vi "CREA_CLUSTER.vi"(0 "FOTOCELULA":bool, 1 "RFID_Error":errorcluster, 4 "RFID_LR6_Error":errorcluster, 6 "DC":bool, 7 "TEMPERATURA":bool, 8 "WHEEL_SENSOR":bool, 9 "all rows":dbl[][](array[numeric]), 10 "LIMITE MAX":dbl, 11 "LIMITE MIN":dbl, 12 "ERROR FPGA":errorcluster, 13 "ERROR ESCRITURA":errorcluster) -> (20 "appended array":cluster{string, dbl, "output string":string}[](array[cluster]), 22 "ESTADO WRD":dbl)   [LabVIEW 2015]
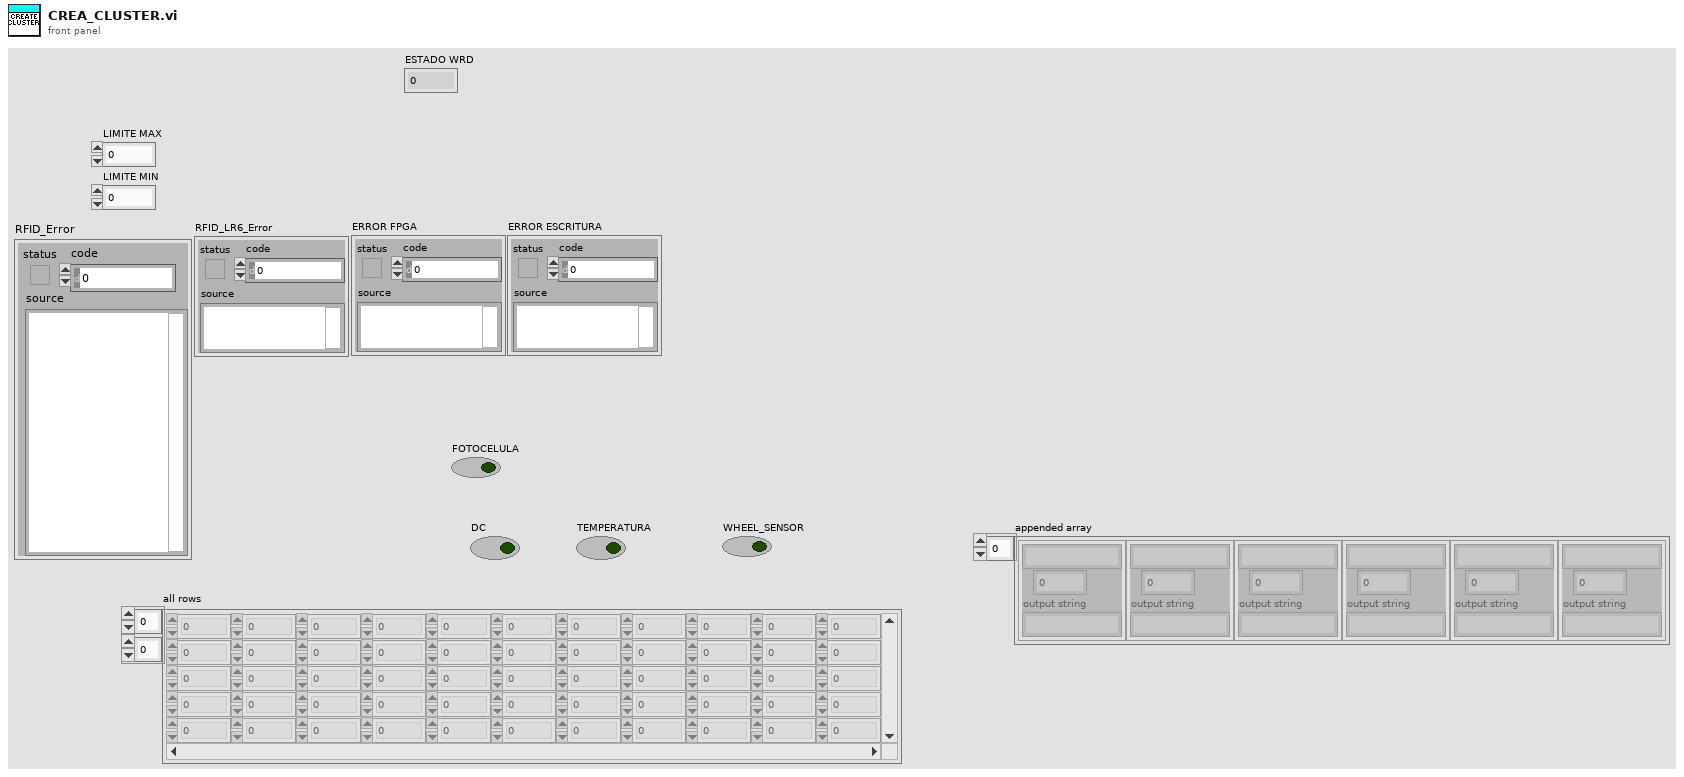
[diagram p1: front panel]
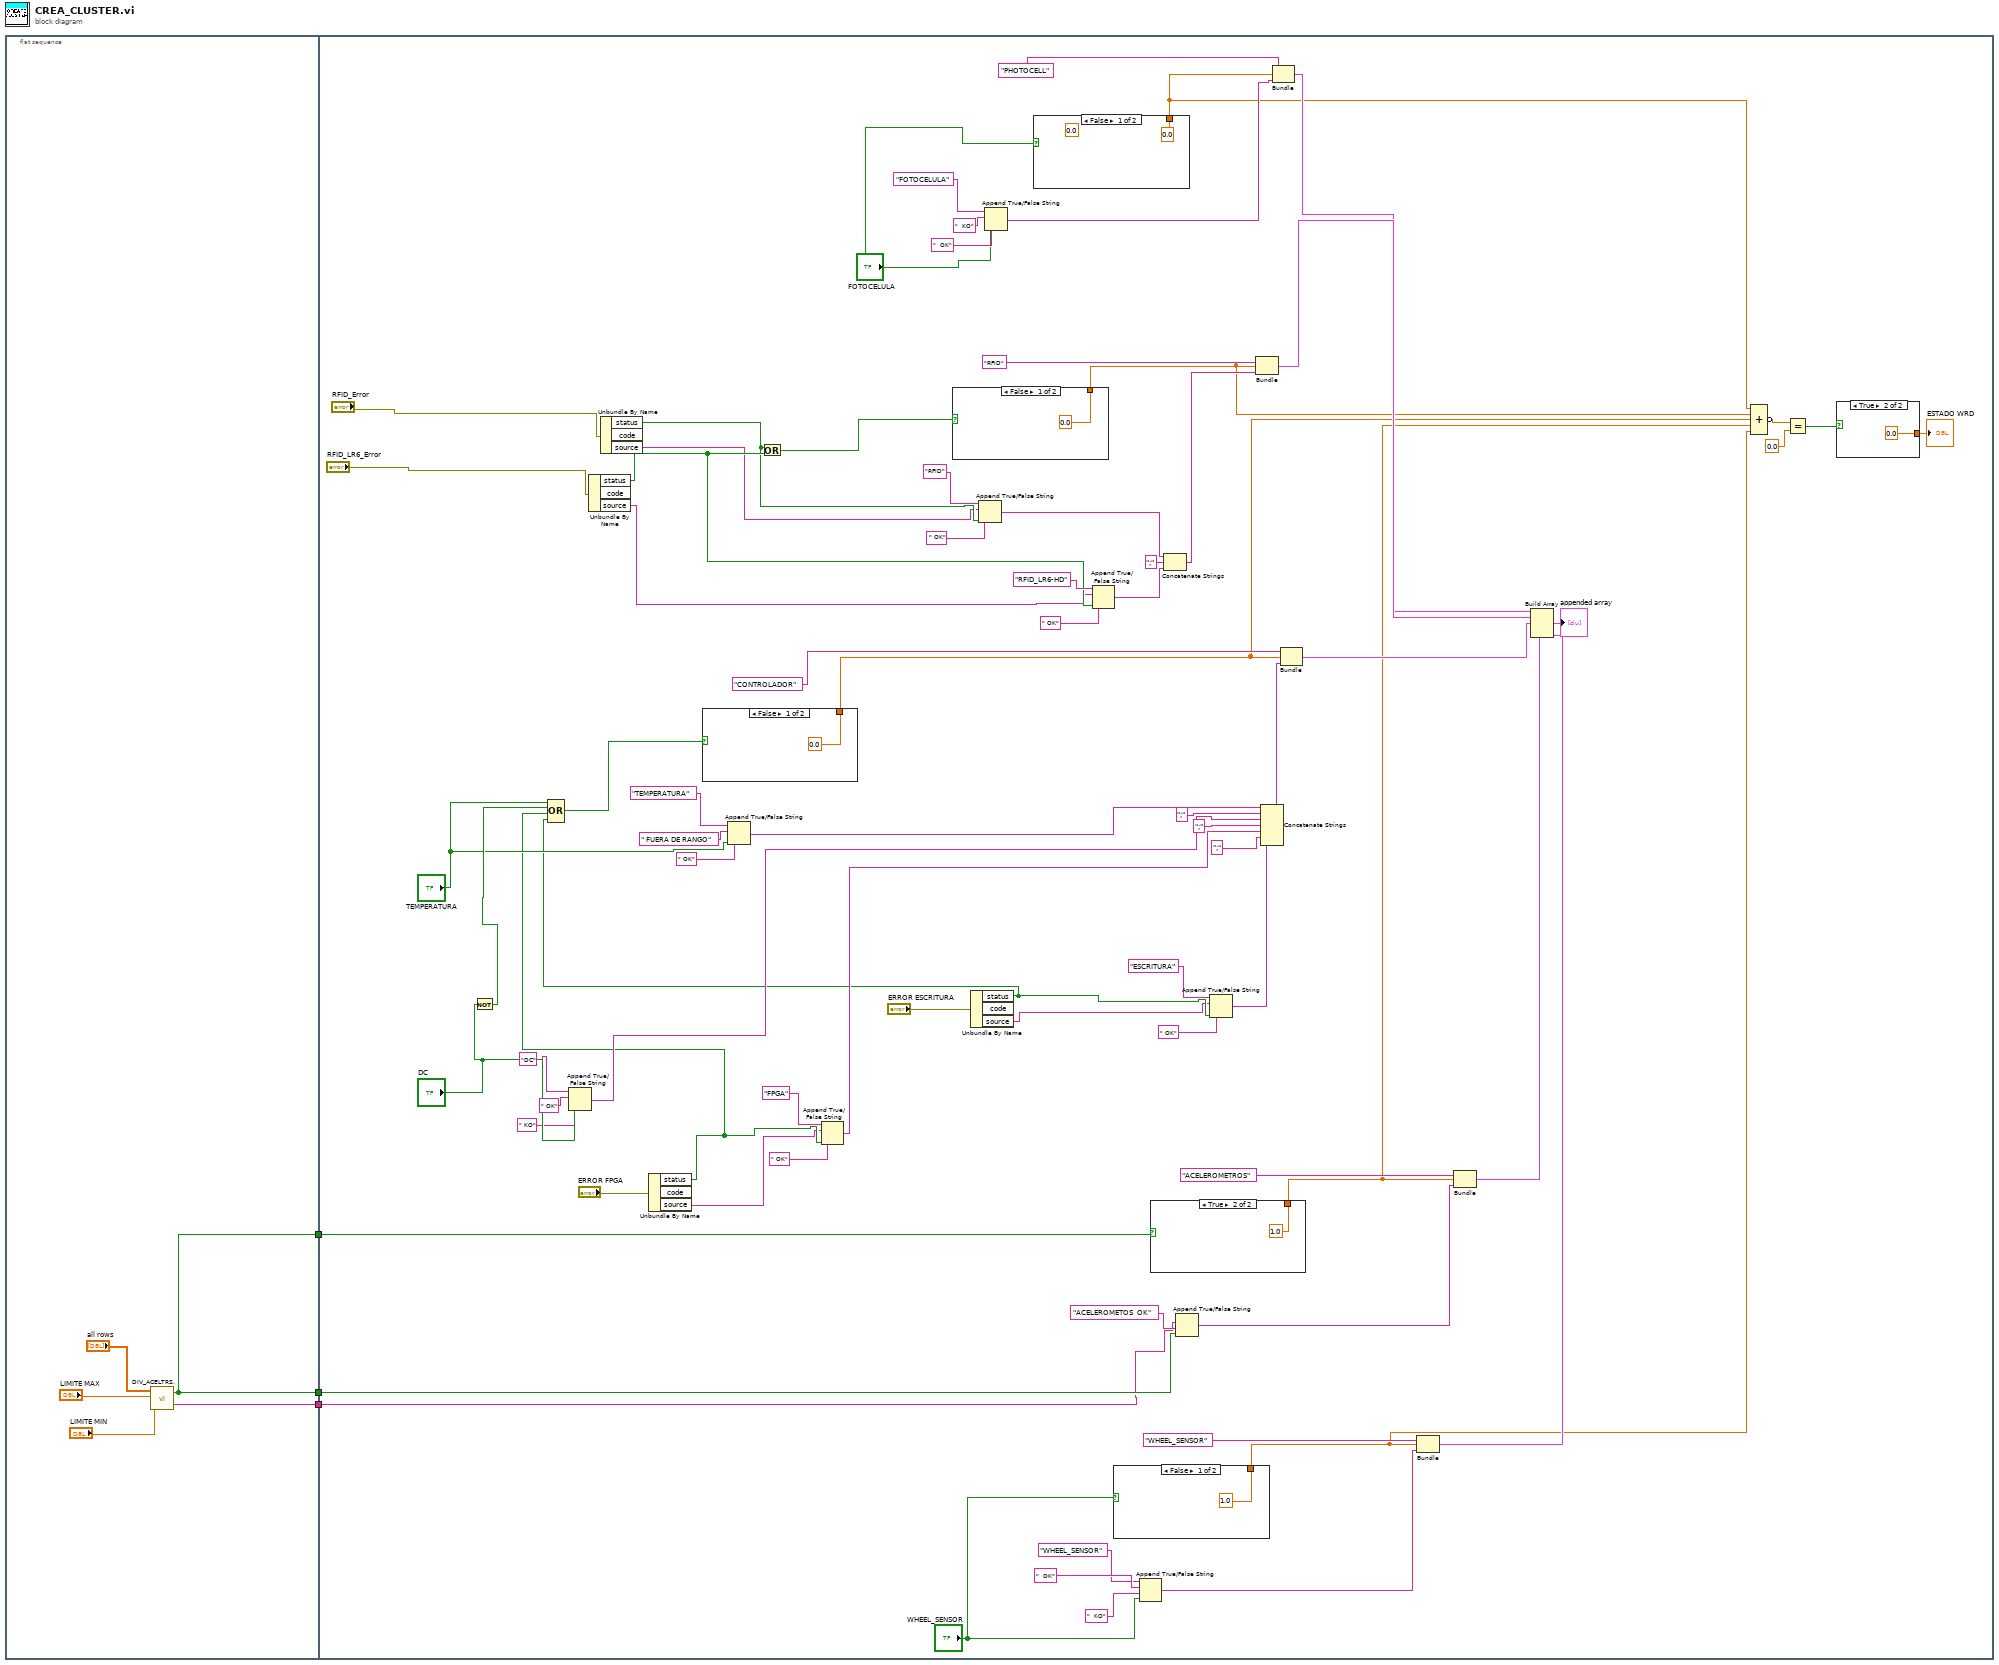
[diagram p0: block diagram]
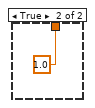
[diagram p2: hidden frame]
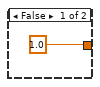
[diagram p3: hidden frame]
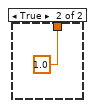
[diagram p4: hidden frame]
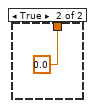
[diagram p5: hidden frame]
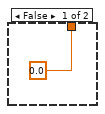
[diagram p6: hidden frame]
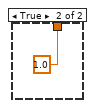
[diagram p7: hidden frame]
diagram:
  n1 = flat-sequence {
    tunnel: [w7] -> w3
    tunnel: [w6] -> w2
    tunnel: [w6] -> w1
    tunnel: w3 -> [w27]
    tunnel: w2 -> [w30]
    tunnel: w1 -> [w35]
    frame #0 {
      n2 = call "DIV_ACELTRS..vi"("LIMITE MIN 2"="LIMITE MIN", "LIMITE MAX 2"="LIMITE MAX", "all rows"="all rows") -> ("concatenated string"=w7:string, "ACELEROMETROS OK"=w6:bool)  [unwired: 3 in]
    }
    frame #1 {
      (unwired) 0.0
      n3 = Not(x="DC") -> (.not. x?=w86:bool)
      n4 = Append True/False String(1:"DC", 2:" KO" ("false string"), 3:" OK" ("true string"), 4:"DC" ("string (\"\")")) -> (0:w80:string)
      n5 = Unbundle By Name("RFID_LR6_Error") -> ("status"=w72:bool, "source"=w17:string)  [unwired: 1 out]
      n6 = Unbundle By Name("RFID_Error") -> ("status"=w71:bool, "source"=w18:string)  [unwired: 1 out]
      n7 = Unbundle By Name("ERROR FPGA") -> ("status"=w10:bool, "source"=w9:string)  [unwired: 1 out]
      n8 = Append True/False String(1:"TEMPERATURA", 2:" OK" ("false string"), 3:" FUERA DE RANGO" ("true string"), 4:"TEMPERATURA" ("string (\"\")")) -> (0:w65:string)
      n9 = Or(x=w71, y=w72) -> (x .or. y?=w73:bool)
      n10 = Append True/False String(1:w10, 2:" OK" ("false string"), 3:w9, 4:"FPGA" ("string (\"\")")) -> (0:w82:string)
      n11 = case shown="False" w73 {
        tunnel: [0.0 1.0] -> w25
        frame False {
        }
        frame True {
        }
      }
      n12 = Unbundle By Name("ERROR ESCRITURA") -> ("status"=w13:bool, "source"=w12:string)  [unwired: 1 out]
      n13 = Compound Arithmetic op=OR("TEMPERATURA", w86, w10, w13) -> (w67:bool)
      n14 = case shown="False" w67 {
        tunnel: [0.0 1.0] -> w24
        frame False {
        }
        frame True {
        }
      }
      n15 = Append True/False String(1:w71, 2:" OK" ("false string"), 3:w18, 4:"RFID" ("string (\"\")")) -> (0:w59:string)
      n16 = Append True/False String(1:"FOTOCELULA", 2:"  OK" ("false string"), 3:"  KO" ("true string"), 4:"FOTOCELULA" ("string (\"\")")) -> (0:w32:string)
      n17 = case shown="False" "FOTOCELULA" {
        tunnel: [0.0 1.0] -> w26
        frame False {
        }
        frame True {
        }
      }
      n18 = Append True/False String(1:w72, 2:" OK" ("false string"), 3:w17, 4:"RFID_LR6-HD" ("string (\"\")")) -> (0:w77:string)
      n19 = case shown="False" "WHEEL_SENSOR" {
        tunnel: [1.0 0.0] -> w22
        frame False {
        }
        frame True {
        }
      }
      n20 = Append True/False String(1:"WHEEL_SENSOR", 2:"  KO" ("false string"), 3:"  OK" ("true string"), 4:"WHEEL_SENSOR" ("string (\"\")")) -> (0:w49:string)
      n21 = case shown="True" w30 {
        tunnel: [0.0 1.0] -> w23
        frame False {
        }
        frame True {
        }
      }
      n22 = Concatenate Strings(w59, ";" ("string"), w77) -> (w60:string)
      n23 = Append True/False String(1:w35, 2:"ACELEROMETOS  OK" ("true string"), 3:w27) -> (0:w44:string)  [unwired: 1 in]
      n24 = Append True/False String(1:w13, 2:" OK" ("false string"), 3:w12, 4:"ESCRITURA" ("string (\"\")")) -> (0:w84:string)
      n25 = Bundle("RFID", w25, w60) -> (w42:cluster{string, dbl, string})  [unwired: 1 in]
      n26 = Concatenate Strings(w65, ";", w80, ";", w82, ";", w84) -> (w66:string)
      n27 = Bundle("PHOTOCELL", w26, "output string"=w32) -> (w31:cluster{string, dbl, "output string":string})  [unwired: 1 in]
      n28 = Bundle("CONTROLADOR", w24, w66) -> (w57:cluster{string, dbl, string})  [unwired: 1 in]
      n29 = Bundle("WHEEL_SENSOR", w22, "output string"=w49) -> (w51:cluster{string, dbl, "output string":string})  [unwired: 1 in]
      n30 = Bundle("ACELEROMETROS", w23, "output string"=w44) -> (w50:cluster{string, dbl, "output string":string})  [unwired: 1 in]
      n31 = Build Array(w31, w42, w57, w50, w51) -> (→"appended array":cluster{string, dbl, "output string":string}[])
      n32 = Compound Arithmetic op=ADD(w26, w25, w24, w23, w22) -> (invert w21:dbl)
      n33 = Equal?(x=w21, y=0.0) -> (x = y?=w19:bool)
      n34 = case shown="True" w19 {
        tunnel: [1.0 0.0] -> w75
        frame False {
        }
        frame True {
        }
      }
      "ESTADO WRD" <- w75
    }
  }
